vi "AutoParameterParser.vi"(2 "Parameter String":string) -> (0 "Remaining Parameter String":string, 1 "Parameter":dbl)   [LabVIEW 2019]
doc: "Parses the next argument in an FRC 4265 autonomous sequence string. Also returns the remainder of the parameter string. Stack these VIs together to extract multiple arguments. Assumes that the parameter is a floating point number."
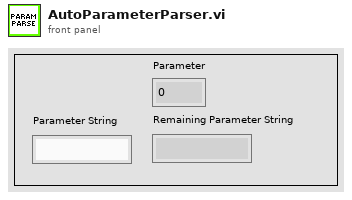
[diagram p1: front panel]
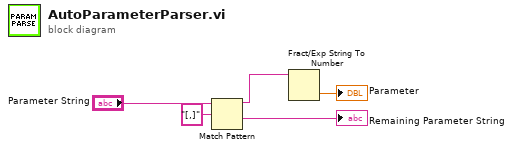
[diagram p0: block diagram]
diagram:
  n1 = Match Pattern(string="Parameter String", regular expression="[,]") -> (before substring=w2:string, after substring=→"Remaining Parameter String":string)  [unwired: 1 in, 2 out]
  n2 = Fract/Exp String To Number(string=w2) -> (number=→"Parameter":dbl)  [unwired: 3 in, 1 out]
